vi "Init.vi"(8 "error in":errorcluster, 11 "Flags":i32 format="%.0x") -> (0 "error out":errorcluster, 3 "Flags Successfully Initialised":i32 format="%.0x")   [LabVIEW 2015, in "LibSDL2_Image.lvlib"]
uses:
  LibSDL2_Image.lvlib
  LibSDL2 Wrapper/DLL/SDL2_image.dll
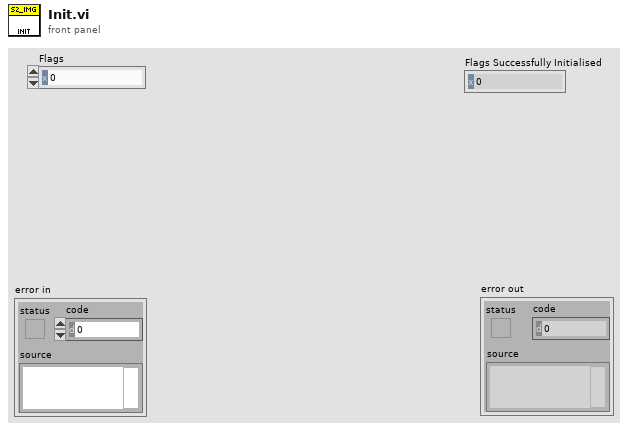
[diagram p1: front panel]
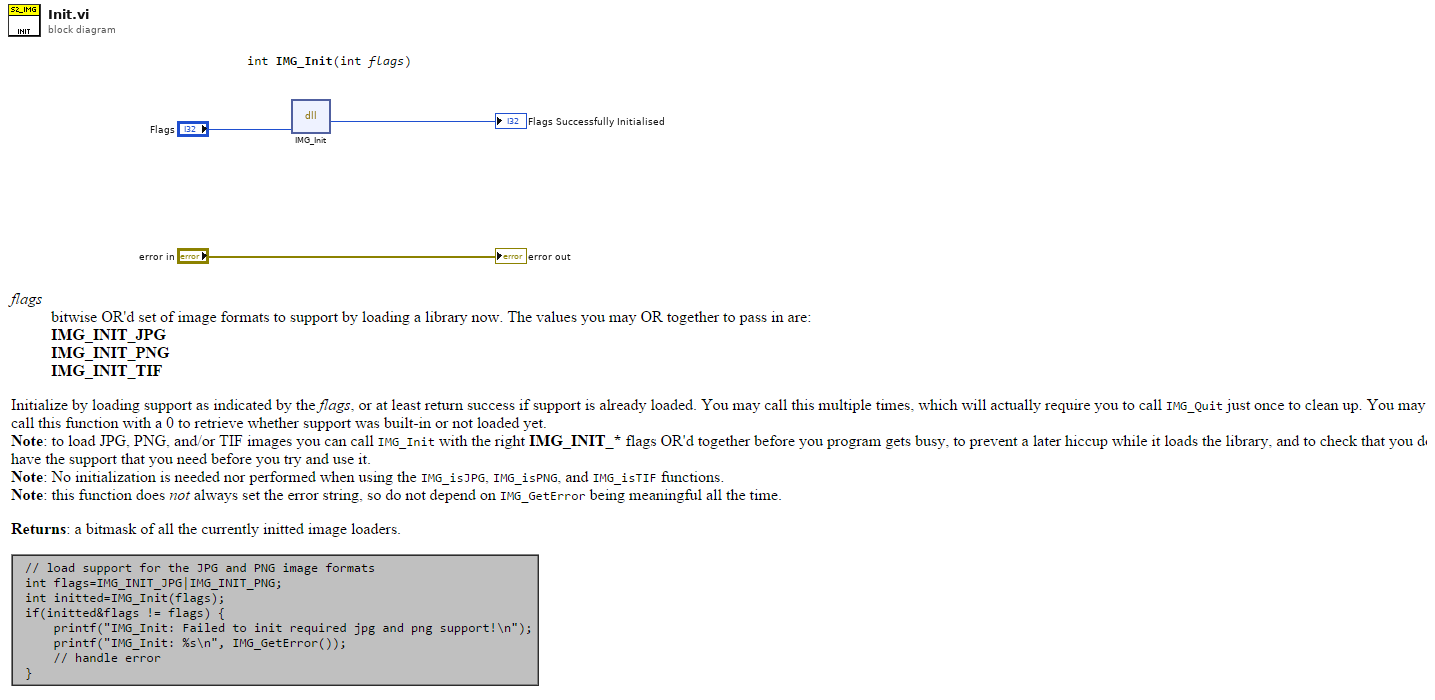
[diagram p0: block diagram]
diagram:
  n1 = dll-call lib="C:/dev/PGS/LabSDL2/Source/Libraries/LibSDL2 Wrapper/DLL/SDL2_image.dll" fn="IMG_Init"("flags"="Flags") -> ("return type"=→"Flags Successfully Initialised":i32)  [unwired: 4 in, 2 out]
  "error out" <- "error in"
